vi "User Console - Transaction to Enum.vi"(8 "error in (no error)":errorcluster, 11 "Transactions":T2) -> (0 "error out":errorcluster, 3 "Transaction Enum":T1)   [LabVIEW 2017]
uses:
  Controls/User Console - Transactions.ctl
  Controls/User Console - Transaction Enum.ctl
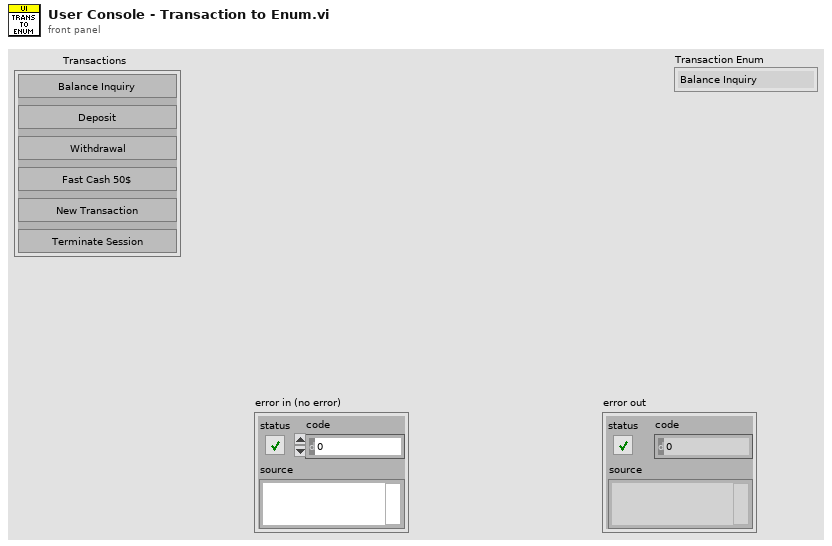
[diagram p1: front panel]
types:
  T1 = typedef "User Console - Transaction Enum.ctl" = enum16{"Balance Inquiry", "Deposit", "Withdrawal", "Fat Cash", "New Transaction", "Terminate Session"}
  T2 = typedef "User Console - Transactions.ctl" = cluster{"Balance Inquiry":bool, "Deposit":bool, "Withdrawal":bool, "Fast Cash":bool, "New Transaction":bool, "Terminate":bool}
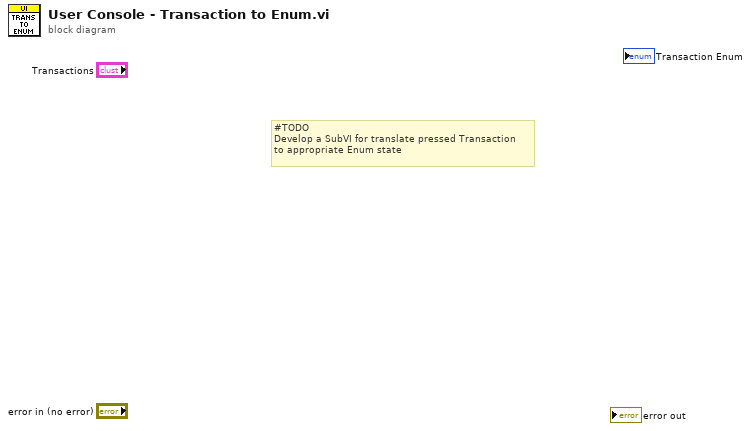
[diagram p0: block diagram]
diagram:
  # "#TODO\nDevelop a SubVI for translate pressed Transaction\nto appropriate Enum state"
